vi "VIs_Start.vi"() -> ()   [LabVIEW 2022 SP3]
panel:
  in  "Temperature Data Collection":path
  in  "Thrust Data Collection":path
  out "error out":errorcluster
  in  "error in (no error)":errorcluster
  in  "cDAQ":path
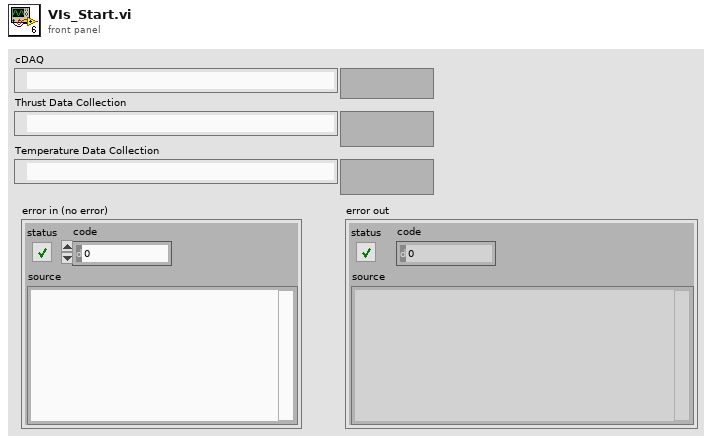
[diagram p1: front panel]
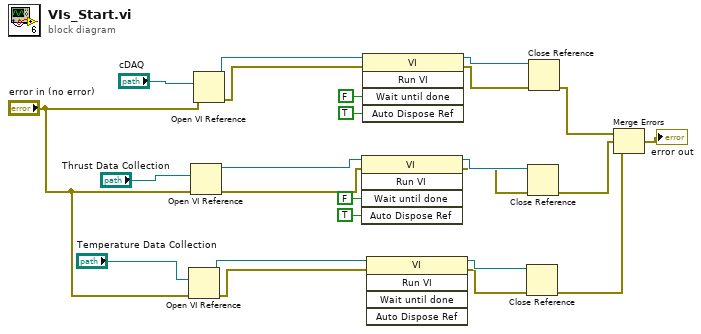
[diagram p0: block diagram]
diagram:
  n1 = Open VI Reference(vi path="Temperature Data Collection", error in (no error)="error in (no error)") -> (vi reference=w4:refnum<vi>, error out=w5:errorcluster)  [unwired: 4 in]
  n2 = Open VI Reference(vi path="Thrust Data Collection", error in (no error)="error in (no error)") -> (vi reference=w21:refnum<vi>, error out=w20:errorcluster)  [unwired: 4 in]
  n3 = Open VI Reference(vi path="cDAQ", error in (no error)="error in (no error)") -> (vi reference=w22:refnum<vi>, error out=w23:errorcluster)  [unwired: 4 in]
  n4 = invoke class="VI" method="Run VI"(reference=w21, error in=w20, "Wait until done"=FALSE ("Wait Until Done"), "Auto Dispose Ref"=TRUE ("Auto Dispose Reference")) -> (reference out=w17:refnum<vi>, error out=w16:errorcluster)  [unwired: 1 in, 3 out]
  n5 = invoke class="VI" method="Run VI"(reference=w22, error in=w23, "Wait until done"=FALSE ("Wait Until Done"), "Auto Dispose Ref"=TRUE ("Auto Dispose Reference")) -> (reference out=w19:refnum<vi>, error out=w18:errorcluster)  [unwired: 1 in, 3 out]
  n6 = invoke class="VI" method="Run VI"(reference=w4, error in=w5) -> (reference out=w3:refnum<vi>, error out=w2:errorcluster)  [unwired: 3 in, 3 out]
  n7 = Close Reference(reference=w3, error in (no error)=w2) -> (error out=w1:errorcluster)
  n8 = Close Reference(reference=w17, error in (no error)=w16) -> (error out=w15:errorcluster)
  n9 = Close Reference(reference=w19, error in (no error)=w18) -> (error out=w14:errorcluster)
  n10 = Merge Errors(w14, w15, w1) -> (→"error out":errorcluster)
